vi "GenerateOuputSequenceList.vi"(11 "input parameters":T1(array[cluster])) -> (1 "output Names":string[](array[string]), 3 "output array":dbl[][](array[numeric]))   [LabVIEW 2015, in "Sequences.lvlib"]
uses:
  Sequences.lvlib
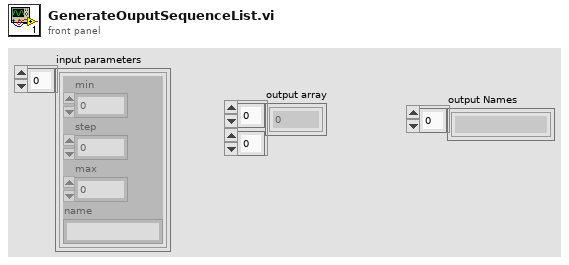
[diagram p1: front panel]
types:
  T1 = cluster{"min":dbl, "step":dbl, "max":dbl, "name":string}[]
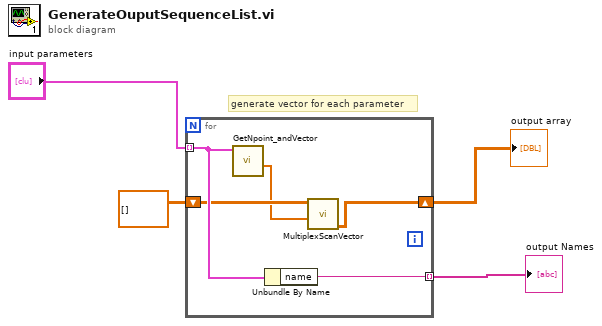
[diagram p0: block diagram]
diagram:
  # "generate vector for each parameter"
  n1 = for {
    tunnel: "input parameters" -> [w8] mode=indexing
    tunnel: [w9] -> w1 mode=indexing
    shift-right: [w7] -> w2
    shift-left: dbl[][] [] ("output array") -> [w6]
    n2 = call "GetNpoint_andVector.vi"("cluster IN"=w8) -> ("Point Array"=w5:dbl[])  [unwired: 9 in, 1 out]
    n3 = Unbundle By Name(w8) -> ("name"=w9:string)
    n4 = call "MultiplexScanVector.vi"("multiplyer"=w5, "initial matrix"=w6) -> ("output array"=w7:dbl[][])  [unwired: 9 in]
  }
  "output array" <- w2
  "output Names" <- w1
